vi "NapovedaEMG(subVI).vi"() -> ()   [LabVIEW 2026]
panel:
  in  "Close":bool
  # "1. Před nalepením elektrod se ujistěte, že je kůže v místech, kam budete nalepovat elektrody, čistá a pokud možno \n    bez ochlupení. Pro lepší vodivost otřete kůži navlhčeným nebo alkoholovým ubrouskem.\n2. Vybalte a nalepte na dobrovolníka elektrody na zvolený sval (např. biceps nebo předloktí). \n    Dvě měřicí elektrody se lepí cca 2 cm od sebe.\n3. Označení elektrod je na PLUX BITalino následující:\n        - černá a červená: měřicí elektrody (nalepte obě na bříško sledovaného svalu).\n        - bílá: referenční elektroda (nalepte na neutrální místo, kde je kost těsně pod kůží – např. loket nebo zápěstí).\n4. Na nalepené elektrody nacvakněte kabely od PLUX BITalina.\n5. Kabel s elektrodami připojte do propojky s nápisem EMG do portu, u kterého není nápis EMG.\n6. Do propojky k nápisu EMG zapojte propojovací kabel a jeho druhý konec do portu A3.\n7. Zapněte PLUX BITalino (LED musí pulsovat).\n8. Spusťte měření."
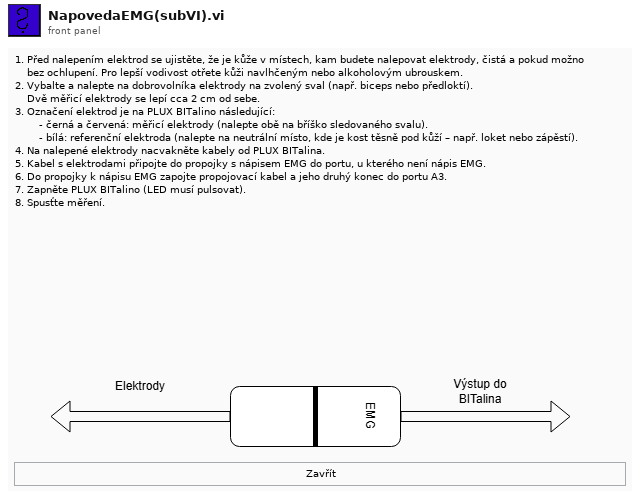
[diagram p1: front panel]
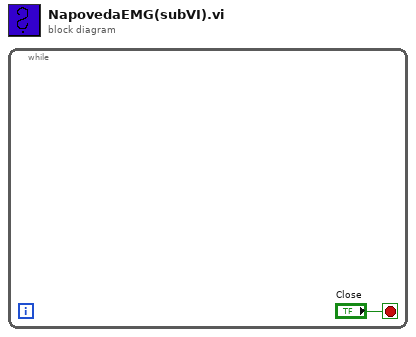
[diagram p0: block diagram]
diagram:
  n1 = while {
    stop <- "Close" stop-if-true
  }
